vi "Conn_vars.vi"(8 "UDPConn In":refnum<k16>, 9 "TCP Conn In":refnum<k5>, 10 "Connected_In":bool, 11 "WriteVars?":bool) -> (0 "Connected_Out":bool, 1 "UDPConnOut":refnum<k16>, 3 "TCPConnOut":refnum<k5>)   [LabVIEW 2014]
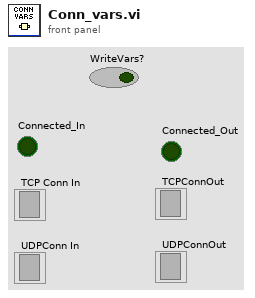
[diagram p1: front panel]
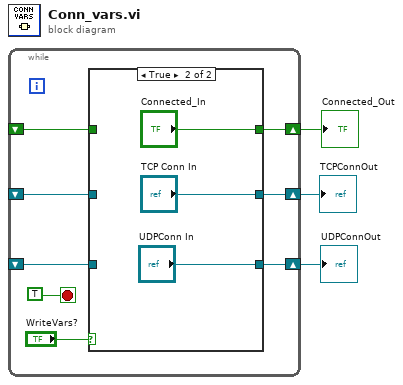
[diagram p0: block diagram]
diagram:
  n1 = while {
    shift-right: [w10] -> w3
    shift-left: _ -> [w7]
    shift-right: [w9] -> w2
    shift-left: _ -> [w6]
    shift-right: [w5] -> w1
    shift-left: _ -> [w4]
    stop <- TRUE stop-if-true
    n2 = case shown="True" "WriteVars?" {
      tunnel: [w14 "TCP Conn In"] -> w10
      tunnel: [w13 "UDPConn In"] -> w9
      tunnel: w7 -> [w14 _]
      tunnel: w6 -> [w13 _]
      tunnel: [w12 "Connected_In"] -> w5
      tunnel: w4 -> [w12 _]
      frame False {
      }
      frame True {
      }
    }
  }
  "TCPConnOut" <- w3
  "UDPConnOut" <- w2
  "Connected_Out" <- w1
